vi "peak detector.vi"(9 "data index":u16, 10 "output valid in":bool, 11 "fft_output":u64) -> (0 "output valid":bool, 1 "adress":u16, 2 "amplitude":u32, 3 "peak":bool)   [LabVIEW 2021]
uses:
  <vilib>/rvi/FXPMathLib/FxpRectToPolar/subVIs/nifxpmath_RectToPolar_SimConfig.ctl
  <vilib>/rvi/FXPMathLib/FxpRectToPolar/simVIs/DllFxpRectToPolarTemp_sub.vi
  <vilib>/rvi/Memory/Memory_Emulation/nirvimemoryFastEmulation.vi
  <vilib>/rvi/Memory/Memory_Emulation/nirvimemoryEmulation.vi
  <vilib>/rvi/Emulation/niFpgaEmulationIsFPGAContextNoSignature.vi
  <vilib>/rvi/DataTransferAndStorage/Container/Common/niFpgaContainerGetUniqueNameForEmu.vi
  <vilib>/rvi/Emulation/niFpgaProcessEmulError.vi
  <vilib>/rvi/Emulation/niFpgaSctlEmulationGetInTimedLoop.vi
  <vilib>/rvi/errors/nirviReportUnexpectedCaseInternalError (U32).vi
  <vilib>/rvi/FXPMathLib/FxpRectToPolar/XNode/nifxpmath_RectToPolar.xnode
  <vilib>/rvi/DataTransferAndStorage/Container/XNode/niFpgaContainer.xnode
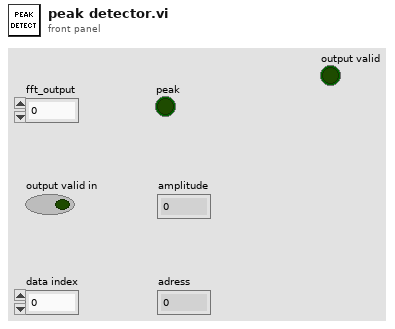
[diagram p1: front panel]
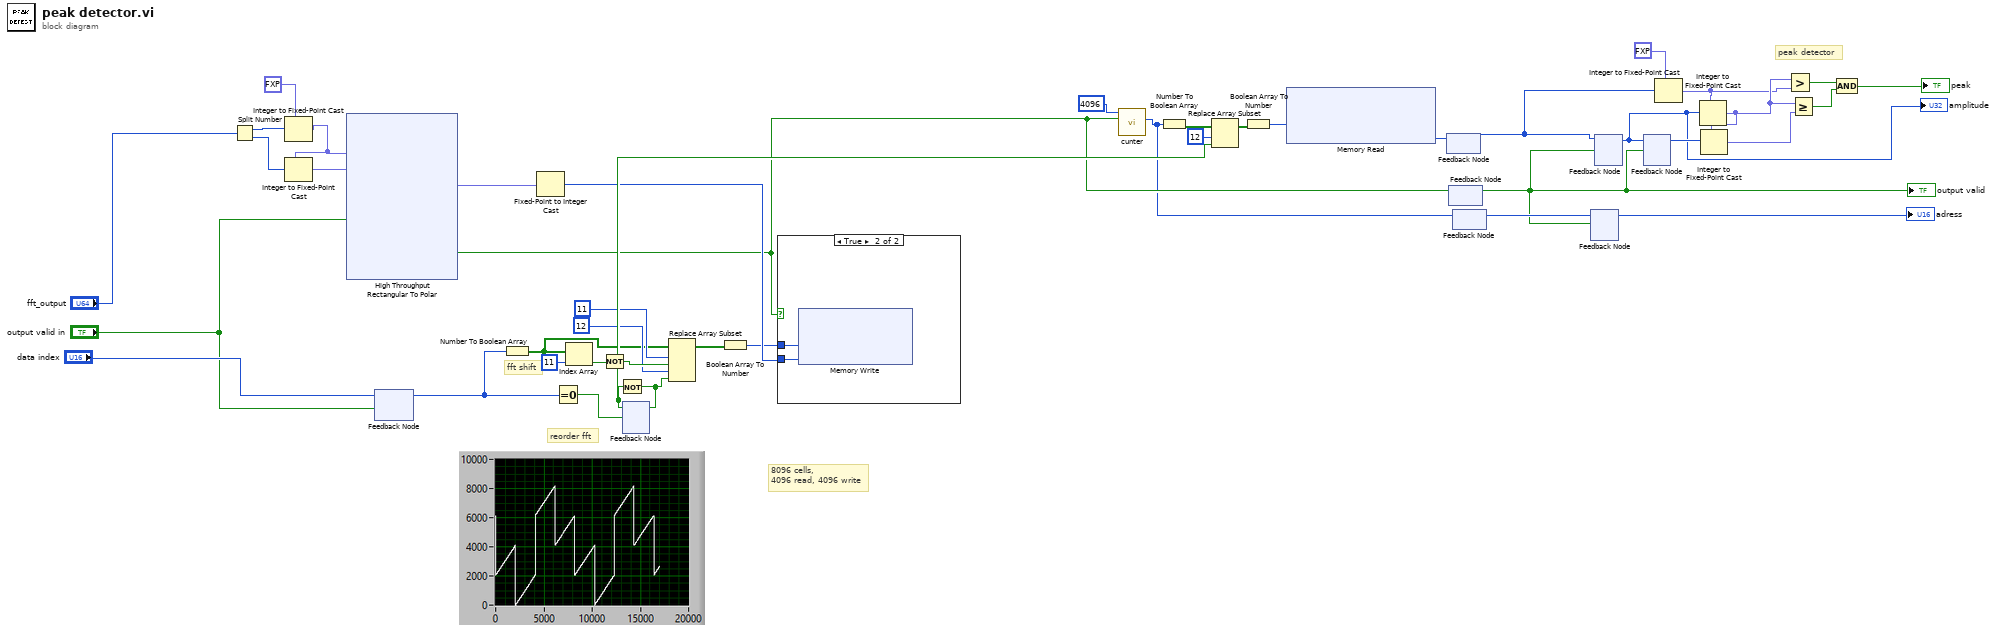
[diagram p0: block diagram]
diagram:
  # "8096 cells,\n4096 read, 4096 write"
  # "reorder fft"
  # "peak detector"
  # "fft shift"
  n1 = Split Number(x="fft_output") -> (hi(x)=w16:u32, lo(x)=w17:u32)
  n2 = Integer to Fixed-Point Cast(fixed-point type=fxp<+/-,32,31> 0.0 ("I"), integer=w16) -> (fixed-point=w19:fxp<+/-,32,31>)
  n3 = Integer to Fixed-Point Cast(fixed-point type=w19, integer=w17) -> (fixed-point=w18:fxp<+/-,32,31>)
  n4 = xnode "High Throughput Rectangular To Polar"("x"=w19, "y"=w18, "input valid"="output valid in") -> ("magnitude"=w33:fxp<+,32,31>, "output valid"=w4:bool)  [unwired: 1 in, 2 out]
  n5 = feedback #1() -> (w31:u16)  [unwired: 1 in]
  n6 = feedback-in #1("data index", "output valid in") -> ()
  n7 = Number To Boolean Array(number=w31) -> (Boolean array=w22:bool[])
  n8 = Fixed-Point to Integer Cast(1:w33) -> (0:w34:u32)
  n9 = Equal To 0?(x=w31) -> (x = 0?=w26:bool)
  n10 = Index Array(array=w22, index=11) -> (element=w21:bool)
  n11 = Not(x=w21) -> (.not. x?=w27:bool)
  n12 = feedback #2() -> (w41:bool)  [unwired: 1 in]
  n13 = Not(x=w41) -> (.not. x?=w28:bool)
  n14 = feedback-in #2(w28, w26) -> ()
  n15 = Replace Array Subset(array=w22, new element #1=w27, index #1=11 ("index"), new element #2=w28, index #2=12 ("index")) -> (w29:bool[])
  n16 = Boolean Array To Number(Boolean array=w29) -> (number=w32:u16)
  n17 = case shown="True" w4 {
    tunnel: w32 -> [_ w45]
    tunnel: w34 -> [_ w44]
    frame False {
    }
    frame True {
      n18 = xnode ("Memory Write")("Address"=w45, "Data"=w44) -> ()  [unwired: 1 in, 1 out]
    }
  }
  n19 = call "cunter.vi"("input valid"=w4, "count to"=u16 4096) -> ("count"=w3:u16)  [unwired: 8 in, 1 out]
  n20 = Number To Boolean Array(number=w3) -> (Boolean array=w36:bool[])
  n21 = Replace Array Subset(array=w36, new element=w41, index=12) -> (w37:bool[])
  n22 = Boolean Array To Number(Boolean array=w37) -> (number=w38:u16)
  n23 = xnode ("Memory Read")("Address"=w38) -> ("Data"=w5:u32)  [unwired: 1 in, 1 out]
  n24 = feedback #3() -> (w6:u32)  [unwired: 1 in]
  n25 = feedback-in #3(w5) -> ()
  n26 = feedback #4() -> (w1:bool)  [unwired: 1 in]
  "output valid" <- w1
  n27 = feedback-in #4(w4) -> ()
  n28 = feedback #5() -> (w2:u16)  [unwired: 1 in]
  n29 = feedback-in #5(w3) -> ()
  n30 = feedback #6() -> (→"adress":u16)  [unwired: 1 in]
  n31 = feedback-in #6(w2, w1) -> ()
  n32 = feedback #7() -> (w7:u32)  [unwired: 1 in]
  "amplitude" <- w7
  n33 = feedback-in #7(w6, w1) -> ()
  n34 = feedback #8() -> (w11:u32)  [unwired: 1 in]
  n35 = feedback-in #8(w7, w1) -> ()
  n36 = Integer to Fixed-Point Cast(fixed-point type=fxp<+,32,31> 0.0 ("magnitude"), integer=w6) -> (fixed-point=w8:fxp<+,32,31>)
  n37 = Integer to Fixed-Point Cast(fixed-point type=w8, integer=w7) -> (fixed-point=w9:fxp<+,32,31>)
  n38 = Integer to Fixed-Point Cast(fixed-point type=w9, integer=w11) -> (fixed-point=w10:fxp<+,32,31>)
  n39 = Greater?(x=w9, y=w8) -> (0:w13:bool)
  n40 = Greater Or Equal?(x=w9, y=w10) -> (x >= y?=w40:bool)
  n41 = Compound Arithmetic op=AND(w13, w40) -> (→"peak":bool)
